vi "报表查询.vi"(11 "ConnectString":string="\"Provider=Microsoft.Jet.OLEDB.4.0;Data Source=C:\\\\Users\\\\Public\\\\Documents\\\\National \n\nInstruments\\\\TestStand 2017 (32-bit)\\\\Components\\\\Models\\\\TestStand Results.mdb;Persist Security Info=False\"") -> ()   [LabVIEW 2018, in "TestStand Simple UI.lvlib"]
uses:
  TestExec.llb/TestStand Simple UI.lvlib
  <vilib>/addons/database/Connection.llb/Conn ObjectReference.ctl
  <vilib>/addons/database/Connection.llb/DB Tools Open Connec (String).vi
  <vilib>/addons/database/Connection.llb/Conn Execute.vi
  <vilib>/addons/database/Recordset.llb/Rec Fetch Recordset Data (R).vi
  <vilib>/addons/database/Recordset.llb/Rec Destroy - Connection.vi
  <vilib>/Utility/file.llb/Write Delimited Spreadsheet (string).vi
  <vilib>/addons/database/_DB Variant To Data/Database Variant To Data.xnode
  <vilib>/addons/database/NI_Database_API.lvlib
panel:
  out "connection reference":T1
  out "error out":errorcluster
  in  "预览":bool
  in  "保存按钮":bool
  in  "搜索按钮":bool
  in  "二维码":string
  out "SN":string
  out "Row":i32
  in  "筛选结果":i32(listbox)
  in  "步骤结果":i32(listbox)
  in  "关键步骤":i32(listbox)
  out "data 2":string[][](array[string])
  out "tables":string[](array[string])
  in  "预览数据":i32(listbox)
  out "data 6":string[][](array[string])
  out "data 5":string[][](array[string])
  out "data 4":string[][](array[string])
  out "data 3":string[][](array[string])
  in  "测试报表":i32(listbox)
  out "data":string[][](array[string])
  in  "树形":string(tree)
  # "测试报表查询"
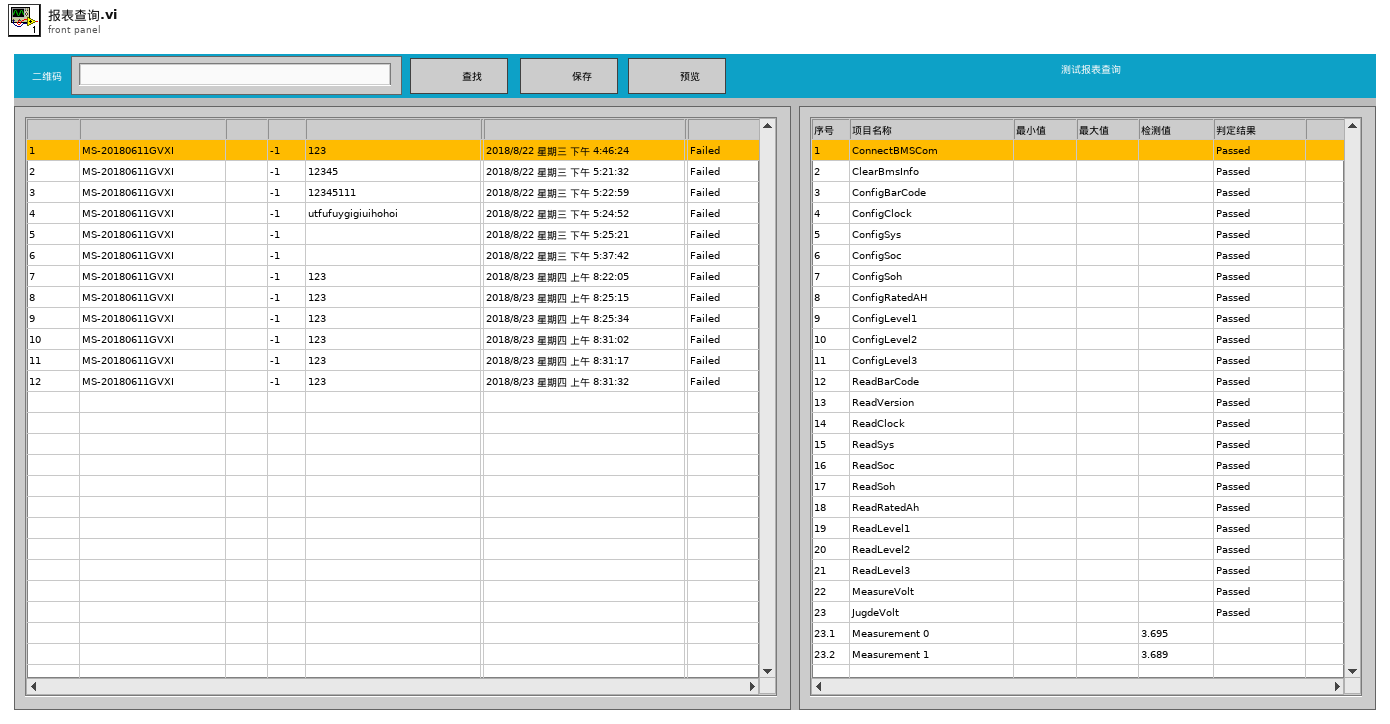
[diagram p1: front panel]
types:
  T1 = typedef "NI_Database_API.lvlib/Conn ObjectReference.ctl" = refnum<k1>
  T2 = typedef "LVPoint32TypeDef.ctl" = cluster{"Horizontal":i32, "Vertical":i32}
  T3 = typedef "LVRowAndColumnTypeDef.ctl" = cluster{"Row":i32, "Column":i32}
  T4 = typedef "NI_Database_API.lvlib/Rec ObjectReference.ctl" = refnum<k1>
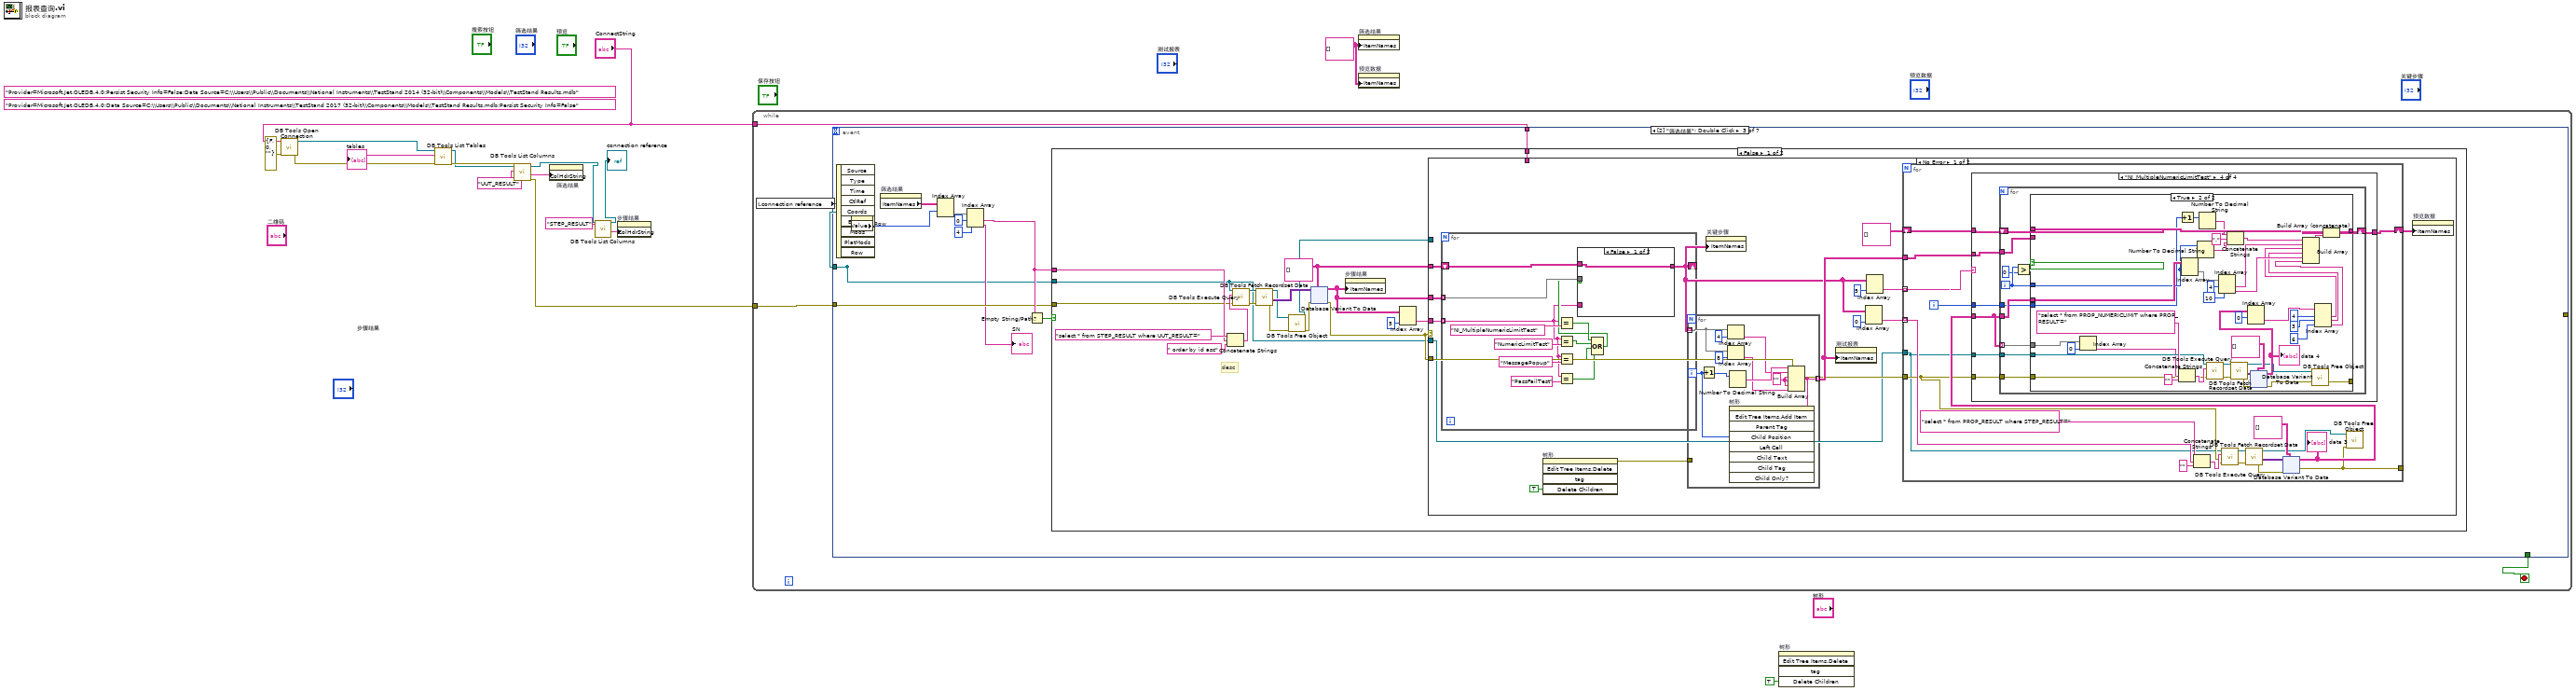
[diagram p0: block diagram]
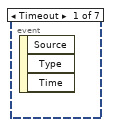
[diagram p2: hidden frame]
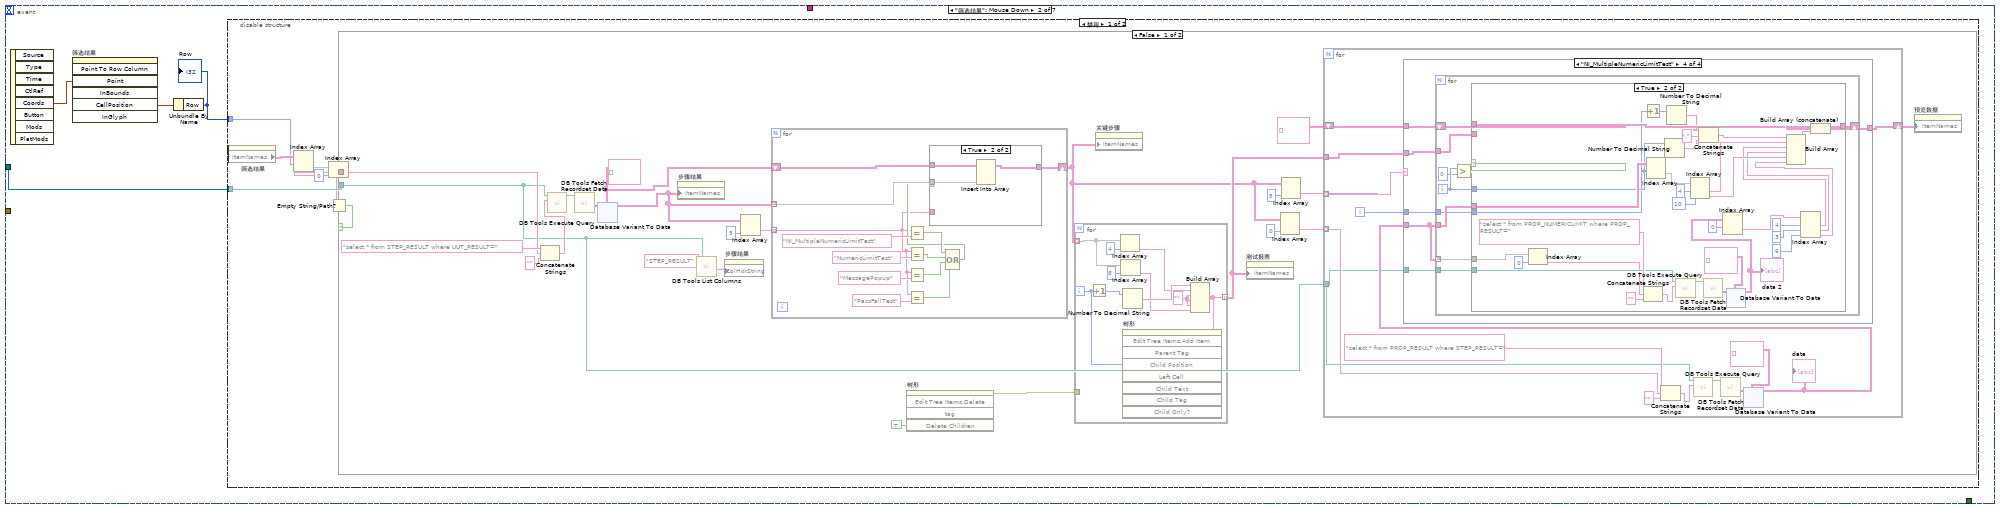
[diagram p3: hidden frame]
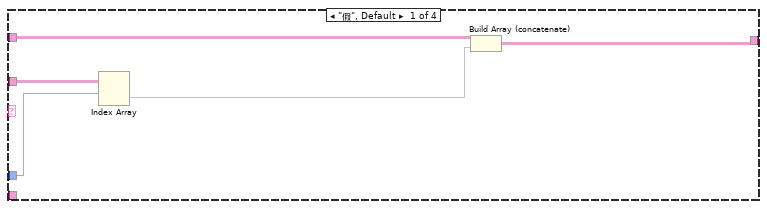
[diagram p4: hidden frame]
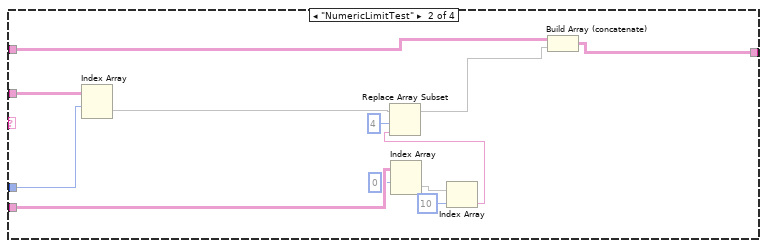
[diagram p5: hidden frame]
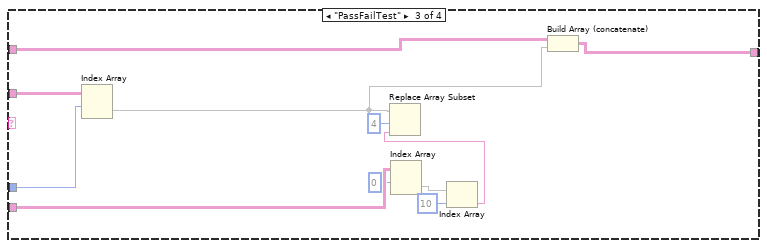
[diagram p6: hidden frame]
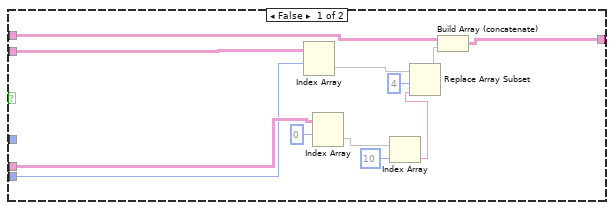
[diagram p7: hidden frame]
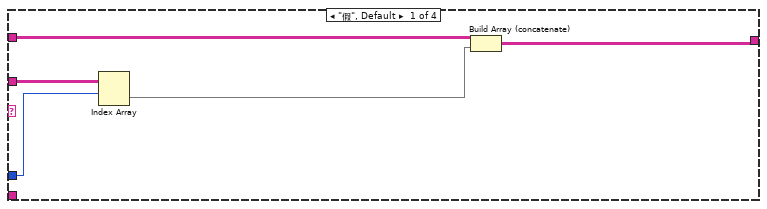
[diagram p11: hidden frame]
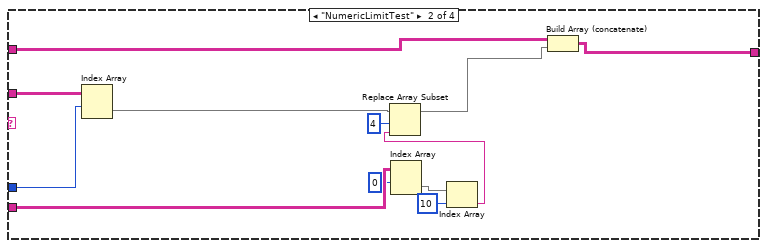
[diagram p12: hidden frame]
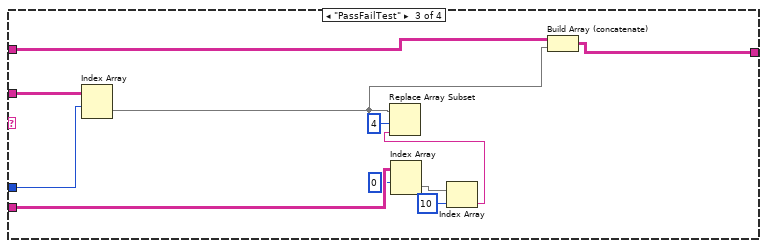
[diagram p13: hidden frame]
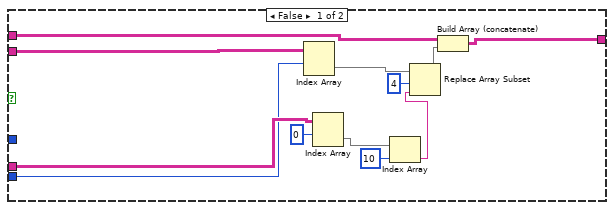
[diagram p14: hidden frame]
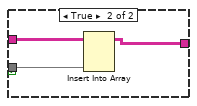
[diagram p15: hidden frame]
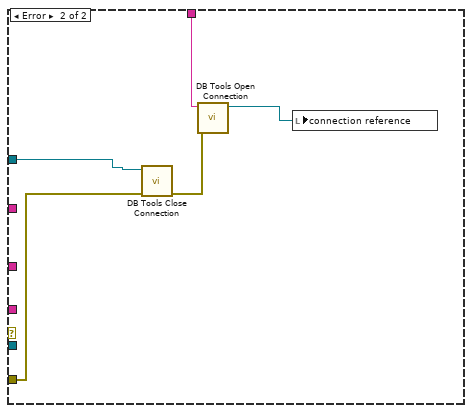
[diagram p16: hidden frame]
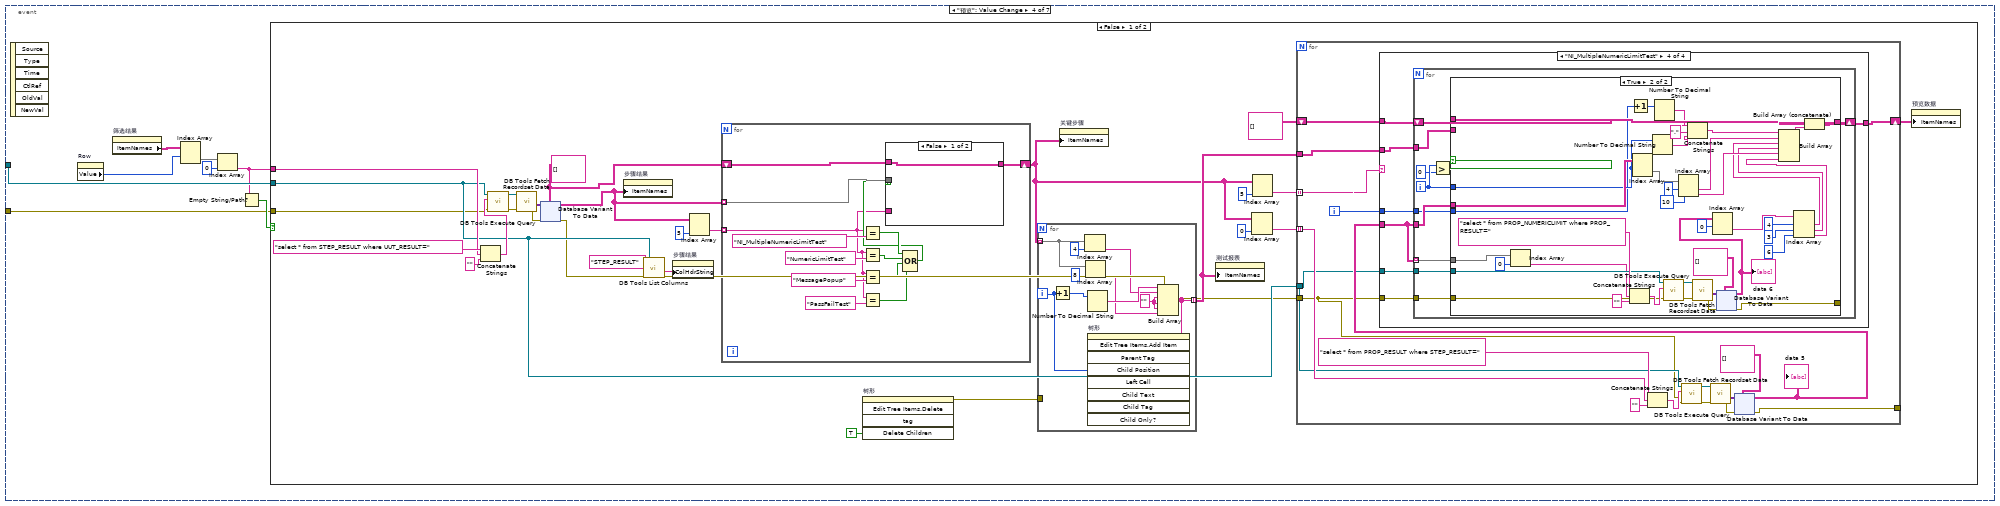
[diagram p18: hidden frame]
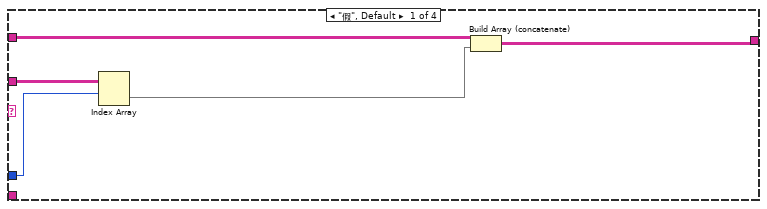
[diagram p19: hidden frame]
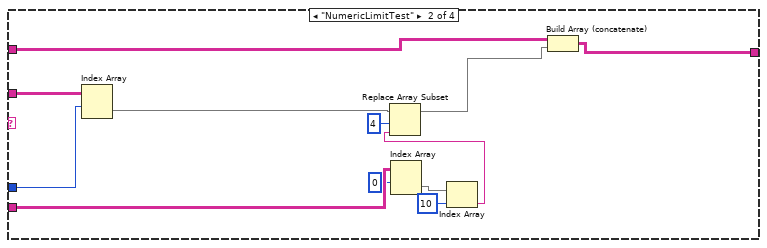
[diagram p20: hidden frame]
diagram:
  w1 = string[][] [] ("Item Names")
  (unwired) "Provider=Microsoft.Jet.OLEDB.4.0;Persist Security Info=False;Data Source=C:\\Users\\Public\\Documents\\National Instruments\\TestStand 2014 (32-bit)\\Components\\Models\\TestStand Results.mdb"
  (unwired) "Provider=Microsoft.Jet.OLEDB.4.0;Data Source=C:\\Users\\Public\\Documents\\National Instruments\\TestStand 2017 (32-bit)\\Components\\Models\\TestStand Results.mdb;Persist Security Info=False"
  n1 = call-poly <vilib>:"DB Tools Open Connection.vi"("error in (no error)"=errorcluster {"status"=FALSE, "code"=0, "source"=""}, "connection information"="ConnectString") -> ("error out"=w10:errorcluster, "connection reference"=w13:T1)  [unwired: 6 in]
  n2 = call <vilib>:"DB Tools List Tables.vi"("error in (no error)"=w10, "connection reference"=w13) -> ("error out"=w9:errorcluster, "tables"=→"tables":string[], "connection reference out"=w7:T1)  [unwired: 3 in]
  n3 = call <vilib>:"DB Tools List Columns.vi"("error in (no error)"=w9, "table"="UUT_RESULT", "connection reference"=w7) -> ("error out"=w8:errorcluster, "columns"=w14:string[], "connection reference out"=w4:T1)  [unwired: 1 in, 1 out]
  n4 = property on="筛选结果" class="MCListbox (strict)"("ColHdrString"=w14) -> ()  [unwired: 2 in, 2 out]
  n5 = call <vilib>:"DB Tools List Columns.vi"("table"="STEP_RESULT", "connection reference"=w4) -> ("columns"=w6:string[], "connection reference out"=→"connection reference":T1)  [unwired: 2 in, 2 out]
  n6 = property on="步骤结果" class="MCListbox (strict)"("ColHdrString"=w6) -> ()  [unwired: 2 in, 2 out]
  n7 = while {
    tunnel: w8 -> [w20]
    tunnel: "ConnectString" -> [w18]
    stop <- w19 stop-if-true
    n8 = local read "connection reference"() -> (w17:T1)
    n9 = event shown="[2] \"筛选结果\": Double Click" {
      selector: _ -> [_ _ _ _ _ _ _]
      dyn-events: _ -> [_ _ _ _ _ _ _]
      timeout: _ -> [_ _ _ _ _ _ _]
      tunnel: w17 -> [_ w22 w319 w649 _ w968 w973]
      tunnel: w20 -> [_ _ w323 w645 _ w967 w971]
      tunnel: [_ _ _ _ _ w969 _] -> w19
      tunnel: [_ _ _ _ _ _ w970] -> _
      tunnel: w18 -> [_ _ w320 _ _ _ _]
      tunnel: [_ _ w319 _ _ _ _] -> _
      event Timeout {
        n10 = event-data() -> ()  [unwired: 1 in, 3 out]
      }
      event "筛选结果": Mouse Down {
        n11 = event-data() -> ("Coords"=w24:T2)  [unwired: 1 in, 7 out]
        n12 = invoke on="筛选结果" class="MCListbox (严格)" method="Point To Row Column"("Point"=w24) -> ("CellPosition"=w23:T3)  [unwired: 6 in, 6 out]
        n13 = Unbundle By Name(w23) -> ("Row"=w21:i32)
        "Row" <- w21
        n14 = disable-structure shown="禁用" {
          disable-tunnel: w22 -> [w28 _]
          disable-tunnel: w21 -> [w27 _]
          frame Disabled {
            n15 = property on="筛选结果" class="MCListbox (strict)"() -> ("ItemNames"=w31:string[][])  [unwired: 2 in, 2 out]
            n16 = Index Array(array=w31, index (row)=w27) -> (element=w30:string[])  [unwired: 1 in]
            n17 = Index Array(array=w30, index=0 ("索引")) -> (element=w26:string)
            n18 = Empty String/Path?(string/path=w26) -> (empty?=w25:bool)
            n19 = case shown="False" w25 {
              tunnel: w28 -> [w36 _]
              tunnel: w26 -> [w48 _]
              frame False {
                w43 = string[][] []
                n20 = Concatenate Strings("select * from STEP_RESULT where UUT_RESULT=" ("condition"), w48, "" ("字符串")) -> (w50:string)
                n21 = call-poly <vilib>:"DB Tools Execute Query.vi"("SQL query"=w50, "connection reference"=w36) -> ("recordset reference"=w54:T4)  [unwired: 6 in, 1 out]
                n22 = call-poly <vilib>:"DB Tools Fetch Recordset Data.vi"("recordset reference"=w54) -> ("recordset data"=w53:variant[][])  [unwired: 4 in, 2 out]
                n23 = xnode "Database Variant To Data"("database variant"=w53, "type"=w43) -> ("data"=w44:string[][])  [unwired: 1 in, 1 out]
                n24 = property on="步骤结果" class="MCListbox (strict)"("ItemNames"=w44) -> ()  [unwired: 2 in, 2 out]
                n25 = call <vilib>:"DB Tools List Columns.vi"("table"="STEP_RESULT", "connection reference"=w36) -> ("columns"=w47:string[])  [unwired: 2 in, 3 out]
                n26 = property on="步骤结果" class="MCListbox (strict)"("ColHdrString"=w47) -> ()  [unwired: 2 in, 2 out]
                n27 = Index Array(array=w44, index (col)=5 ("禁用的索引 (列)")) -> (element=w45:string[])  [unwired: 1 in]
                n28 = for {
                  tunnel: w45 -> [w259] mode=indexing
                  tunnel: w44 -> [w263] mode=indexing
                  shift-right: [w261] -> w38
                  shift-left: w43 -> [w264]
                  n29 = Equal?(x=w259, y="NI_MultipleNumericLimitTest") -> (x = y?=w267:bool)
                  n30 = Equal?(x=w259, y="NumericLimitTest") -> (x = y?=w266:bool)
                  n31 = Equal?(x=w259, y="MessagePopup") -> (x = y?=w265:bool)
                  n32 = Equal?(x=w259, y="PassFailTest") -> (x = y?=w258:bool)
                  n33 = Compound Arithmetic op=OR(w267, w266, w265, w258) -> (w262:bool)
                  n34 = case shown="True" w262 {
                    tunnel: w264 -> [w271 w274]
                    tunnel: w263 -> [_ w273]
                    tunnel: [w271 w272] -> w261
                    tunnel: w259 -> [_ _]
                    frame False {
                    }
                    frame True {
                      n35 = Insert Into Array(array=w274, new element=w273) -> (w272:string[][])  [unwired: 2 in]
                    }
                  }
                }
                n36 = invoke on="树形" class="Tree (严格)" method="Edit Tree Items.Delete"("Delete Children"=TRUE ("删除子项？")) -> (error out=w34:errorcluster)  [unwired: 4 in, 4 out]
                n37 = for {
                  tunnel: w38 -> [w253] mode=indexing
                  tunnel: [w249] -> w42 mode=indexing
                  tunnel: w34 -> [_]
                  i -> [w248]
                  w251 = ""
                  n38 = Increment(x=w248) -> (x+1=w257:i32)
                  n39 = Index Array(array=w253, index=4 ("索引")) -> (element=w254:string)
                  n40 = Index Array(array=w253, index=8 ("索引")) -> (element=w250:string)
                  n41 = Number To Decimal String(number=w257) -> (decimal integer string=w256:string)  [unwired: 1 in]
                  n42 = Build Array(w256, w254, w251, w251, w251, w250) -> (w249:string[])
                  n43 = invoke on="树形" class="Tree (严格)" method="Edit Tree Items.Add Item"("Child Position"=w248, "Child Text"=w249) -> ()  [unwired: 7 in, 9 out]
                }
                n44 = property on="关键步骤" class="MCListbox (strict)"("ItemNames"=w38) -> ()  [unwired: 2 in, 2 out]
                n45 = property on="测试报表" class="MCListbox (strict)"("ItemNames"=w42) -> ()  [unwired: 2 in, 2 out]
                n46 = Index Array(array=w38, index (col)=0 ("禁用的索引 (列)")) -> (element=w37:string[])  [unwired: 1 in]
                n47 = Index Array(array=w38, index (col)=5 ("禁用的索引 (列)")) -> (element=w40:string[])  [unwired: 1 in]
                n48 = for {
                  tunnel: w40 -> [w68] mode=indexing
                  tunnel: w37 -> [w61] mode=indexing
                  tunnel: w36 -> [w55]
                  shift-right: [w57] -> w32
                  shift-left: string[][] [] -> [w58]
                  tunnel: w42 -> [w60]
                  i -> [w59]
                  n49 = Concatenate Strings("select * from PROP_RESULT where STEP_RESULT=" ("condition"), w61, "" ("字符串")) -> (w64:string)
                  n50 = call-poly <vilib>:"DB Tools Execute Query.vi"("SQL query"=w64, "connection reference"=w55) -> ("recordset reference"=w67:T4)  [unwired: 6 in, 1 out]
                  n51 = call-poly <vilib>:"DB Tools Fetch Recordset Data.vi"("recordset reference"=w67) -> ("recordset data"=w66:variant[][])  [unwired: 4 in, 2 out]
                  n52 = xnode "Database Variant To Data"("database variant"=w66, "type"=string[][] []) -> ("data"=w56:string[][])  [unwired: 1 in, 1 out]
                  "data" <- w56
                  n53 = case shown="\"NI_MultipleNumericLimitTest\"" w68 {
                    tunnel: w60 -> [w116 w122 w134 w142]
                    tunnel: w59 -> [w113 w121 w133 w146]
                    tunnel: w56 -> [_ w127 w139 w144]
                    tunnel: w58 -> [w117 w120 w132 w143]
                    tunnel: [w114 w118 w131 w145] -> w57
                    tunnel: w55 -> [_ _ _ w141]
                    frame "假", Default {
                      n54 = Index Array(array=w116, index (row)=w113) -> (element=w115:string[])  [unwired: 1 in]
                      n55 = Build Array (concatenate)(w117, w115) -> (w114:string[][])
                    }
                    frame "NumericLimitTest" {
                      n56 = Index Array(array=w122, index (row)=w121) -> (element=w129:string[])  [unwired: 1 in]
                      n57 = Index Array(array=w127, index (row)=0 ("索引 (行)")) -> (element=w125:string[])  [unwired: 1 in]
                      n58 = Index Array(array=w125, index=10 ("索引")) -> (element=w123:string)
                      n59 = Replace Array Subset(array=w129, new element=w123, index=4 ("索引")) -> (w119:string[])
                      n60 = Build Array (concatenate)(w120, w119) -> (w118:string[][])
                    }
                    frame "PassFailTest" {
                      n61 = Index Array(array=w134, index (row)=w133) -> (element=w130:string[])  [unwired: 1 in]
                      n62 = Index Array(array=w139, index (row)=0 ("索引 (行)")) -> (element=w137:string[])  [unwired: 1 in]
                      n63 = Index Array(array=w137, index=10 ("索引")) -> (element=w135:string)
                      n64 = Replace Array Subset(array=w130, new element=w135, index=4 ("索引")) -> ()  [unwired: 1 out]
                      n65 = Build Array (concatenate)(w132, w130) -> (w131:string[][])
                    }
                    frame "NI_MultipleNumericLimitTest" {
                      n66 = for {
                        tunnel: w144 -> [w156]
                        tunnel: w142 -> [w155]
                        tunnel: w146 -> [w154]
                        shift-right: [w152] -> w145
                        shift-left: w143 -> [w153]
                        tunnel: w144 -> [w147] mode=indexing
                        tunnel: w141 -> [w148]
                        i -> [w151]
                        n67 = Greater?(x=w151, y=0) -> (0:w150:bool)
                        n68 = case shown="True" w150 {
                          tunnel: w156 -> [w166 w200]
                          tunnel: w155 -> [w168 _]
                          tunnel: w154 -> [w165 w188]
                          tunnel: w153 -> [w159 w202]
                          tunnel: [w157 w201] -> w152
                          tunnel: w151 -> [_ w198]
                          tunnel: w148 -> [_ w181]
                          tunnel: w147 -> [_ w180]
                          frame False {
                            n69 = Index Array(array=w168, index (row)=w165) -> (element=w167:string[])  [unwired: 1 in]
                            n70 = Index Array(array=w166, index (row)=0 ("索引 (行)")) -> (element=w163:string[])  [unwired: 1 in]
                            n71 = Index Array(array=w163, index=10 ("索引")) -> (element=w160:string)
                            n72 = Replace Array Subset(array=w167, new element=w160, index=4 ("索引")) -> (w158:string[])
                            n73 = Build Array (concatenate)(w159, w158) -> (w157:string[][])
                          }
                          frame True {
                            n74 = Index Array(array=w180, index=0 ("索引")) -> (element=w178:string)
                            n75 = Concatenate Strings("select * from PROP_NUMERICLIMIT where PROP_RESULT=" ("condition"), w178, "" ("字符串")) -> (w185:string)
                            n76 = Increment(x=w188) -> (x+1=w189:i32)
                            n77 = Index Array(array=w200, index (row)=w198) -> (element=w199:string[])  [unwired: 1 in]
                            n78 = Number To Decimal String(number=w198) -> (decimal integer string=w191:string)  [unwired: 1 in]
                            n79 = Number To Decimal String(number=w189) -> (decimal integer string=w193:string)  [unwired: 1 in]
                            n80 = call-poly <vilib>:"DB Tools Execute Query.vi"("SQL query"=w185, "connection reference"=w181) -> ("recordset reference"=w182:T4)  [unwired: 6 in, 1 out]
                            n81 = Index Array(array=w199, index #1=4 ("索引"), index #2=10 ("索引")) -> (element #1=w196:string, element #2=w195:string)
                            n82 = Concatenate Strings(w193, "." ("字符串"), w191) -> (w190:string)
                            n83 = call-poly <vilib>:"DB Tools Fetch Recordset Data.vi"("recordset reference"=w182) -> ("recordset data"=w183:variant[][])  [unwired: 4 in, 2 out]
                            n84 = xnode "Database Variant To Data"("database variant"=w183, "type"=string[][] []) -> ("data"=w176:string[][])  [unwired: 1 in, 1 out]
                            "data 2" <- w176
                            n85 = Index Array(array=w176, index (row)=0 ("索引")) -> (element=w175:string[])  [unwired: 1 in]
                            n86 = Index Array(array=w175, index #1=4 ("索引"), index #2=3 ("索引"), index #3=6 ("索引")) -> (element #1=w171:string, element #2=w170:string, element #3=w169:string)
                            n87 = Build Array(w190, w196, w171, w170, w195, w169) -> (w194:string[])
                            n88 = Build Array (concatenate)(w202, w194) -> (w201:string[][])
                          }
                        }
                      }
                    }
                  }
                }
                n89 = property on="预览数据" class="MCListbox (strict)"("ItemNames"=w32) -> ()  [unwired: 2 in, 2 out]
              }
              frame True {
              }
            }
          }
          frame Enabled {
          }
        }
      }
      event "筛选结果": Double Click {
        n90 = event-data() -> ()  [unwired: 1 in, 9 out]
        n91 = property on="Row" class="DigNum (strict)"() -> ("Value"=w324:i32)  [unwired: 2 in, 2 out]
        n92 = property on="筛选结果" class="MCListbox (strict)"() -> ("ItemNames"=w329:string[][])  [unwired: 2 in, 2 out]
        n93 = Index Array(array=w329, index (row)=w324) -> (element=w328:string[])  [unwired: 1 in]
        n94 = Index Array(array=w328, index #1=0 ("索引"), index #2=4 ("索引")) -> (element #1=w326:string, element #2=→"SN":string)
        n95 = Empty String/Path?(string/path=w326) -> (empty?=w325:bool)
        n96 = case shown="False" w325 {
          tunnel: w319 -> [w334 _]
          tunnel: w326 -> [w343 _]
          tunnel: w323 -> [w335 _]
          tunnel: w320 -> [w337 _]
          frame False {
            w339 = string[][] []
            # "desc"
            n97 = Concatenate Strings("select * from STEP_RESULT where UUT_RESULT=" ("condition"), w343, " order by id asc" ("字符串")) -> (w344:string)
            n98 = call-poly <vilib>:"DB Tools Execute Query.vi"("error in (no error)"=w335, "SQL query"=w344, "connection reference"=w334) -> ("error out"=w338:errorcluster, "recordset reference"=w348:T4)  [unwired: 5 in]
            n99 = call-poly <vilib>:"DB Tools Fetch Recordset Data.vi"("error in (no error)"=w338, "recordset reference"=w348) -> ("error out"=w332:errorcluster, "recordset data"=w347:variant[][], "recordset reference out"=w333:T4)  [unwired: 3 in]
            n100 = call-poly <vilib>:"DB Tools Free Object.vi"("error in (no error)"=w332, "recordset reference"=w333) -> ("error out"=w331:errorcluster, "connection reference"=w330:T1)  [unwired: 8 in]
            n101 = xnode "Database Variant To Data"("database variant"=w347, "error in (no error)"=w331, "type"=w339) -> ("data"=w340:string[][], "error out"=w336:errorcluster)
            n102 = property on="步骤结果" class="MCListbox (strict)"("ItemNames"=w340) -> ()  [unwired: 2 in, 2 out]
            n103 = Index Array(array=w340, index (col)=5 ("禁用的索引 (列)")) -> (element=w341:string[])  [unwired: 1 in]
            n104 = case shown="No Error" w336 {
              tunnel: w341 -> [w363 _]
              tunnel: w340 -> [w362 _]
              tunnel: w339 -> [w361 _]
              tunnel: w336 -> [w350 w596]
              tunnel: w337 -> [_ w600]
              tunnel: w334 -> [w349 _]
              tunnel: w330 -> [_ w597]
              frame No Error {
                n105 = for {
                  tunnel: w363 -> [w580] mode=indexing
                  tunnel: w362 -> [w584] mode=indexing
                  shift-right: [w582] -> w356
                  shift-left: w361 -> [w585]
                  n106 = Equal?(x=w580, y="NI_MultipleNumericLimitTest") -> (x = y?=w588:bool)
                  n107 = Equal?(x=w580, y="NumericLimitTest") -> (x = y?=w587:bool)
                  n108 = Equal?(x=w580, y="MessagePopup") -> (x = y?=w586:bool)
                  n109 = Equal?(x=w580, y="PassFailTest") -> (x = y?=w579:bool)
                  n110 = Compound Arithmetic op=OR(w588, w587, w586, w579) -> (w583:bool)
                  n111 = case shown="False" w583 {
                    tunnel: w585 -> [w592 w595]
                    tunnel: w584 -> [_ w594]
                    tunnel: [w592 w593] -> w582
                    tunnel: w580 -> [_ _]
                    frame False {
                    }
                    frame True {
                      n112 = Insert Into Array(array=w595, new element=w594) -> (w593:string[][])  [unwired: 2 in]
                    }
                  }
                }
                n113 = invoke on="树形" class="Tree (严格)" method="Edit Tree Items.Delete"("Delete Children"=TRUE ("删除子项？")) -> (error out=w353:errorcluster)  [unwired: 4 in, 4 out]
                n114 = for {
                  tunnel: w356 -> [w574] mode=indexing
                  tunnel: [w570] -> w360 mode=indexing
                  tunnel: w353 -> [_]
                  i -> [w569]
                  w572 = ""
                  n115 = Increment(x=w569) -> (x+1=w578:i32)
                  n116 = Index Array(array=w574, index=4 ("索引")) -> (element=w575:string)
                  n117 = Index Array(array=w574, index=8 ("索引")) -> (element=w571:string)
                  n118 = Number To Decimal String(number=w578) -> (decimal integer string=w577:string)  [unwired: 1 in]
                  n119 = Build Array(w577, w575, w572, w572, w572, w571) -> (w570:string[])
                  n120 = invoke on="树形" class="Tree (严格)" method="Edit Tree Items.Add Item"("Child Position"=w569, "Child Text"=w570) -> ()  [unwired: 7 in, 9 out]
                }
                n121 = property on="关键步骤" class="MCListbox (strict)"("ItemNames"=w356) -> ()  [unwired: 2 in, 2 out]
                n122 = property on="测试报表" class="MCListbox (strict)"("ItemNames"=w360) -> ()  [unwired: 2 in, 2 out]
                n123 = Index Array(array=w356, index (col)=0 ("禁用的索引 (列)")) -> (element=w355:string[])  [unwired: 1 in]
                n124 = Index Array(array=w356, index (col)=5 ("禁用的索引 (列)")) -> (element=w358:string[])  [unwired: 1 in]
                n125 = for {
                  tunnel: w358 -> [w382] mode=indexing
                  tunnel: w355 -> [w375] mode=indexing
                  tunnel: w349 -> [w364]
                  shift-right: [w371] -> w351
                  shift-left: string[][] [] -> [w372]
                  tunnel: w360 -> [w374]
                  tunnel: w350 -> [w369]
                  tunnel: [w365] -> _
                  i -> [w373]
                  n126 = Concatenate Strings("select * from PROP_RESULT where STEP_RESULT=" ("condition"), w375, "" ("字符串")) -> (w378:string)
                  n127 = call-poly <vilib>:"DB Tools Execute Query.vi"("error in (no error)"=w369, "SQL query"=w378, "connection reference"=w364) -> ("error out"=w368:errorcluster, "recordset reference"=w381:T4)  [unwired: 5 in]
                  n128 = call-poly <vilib>:"DB Tools Fetch Recordset Data.vi"("error in (no error)"=w368, "recordset reference"=w381) -> ("error out"=w367:errorcluster, "recordset data"=w380:variant[][], "recordset reference out"=w366:T4)  [unwired: 3 in]
                  n129 = xnode "Database Variant To Data"("database variant"=w380, "error in (no error)"=w367, "type"=string[][] []) -> ("data"=w370:string[][], "error out"=w365:errorcluster)
                  "data 3" <- w370
                  n130 = case shown="\"NI_MultipleNumericLimitTest\"" w382 {
                    tunnel: w374 -> [w430 w436 w448 w457]
                    tunnel: w373 -> [w427 w435 w447 w461]
                    tunnel: w370 -> [_ w441 w453 w459]
                    tunnel: w372 -> [w431 w434 w446 w458]
                    tunnel: [w428 w432 w445 w460] -> w371
                    tunnel: w364 -> [_ _ _ w456]
                    tunnel: w369 -> [_ _ _ w455]
                    frame "假", Default {
                      n131 = Index Array(array=w430, index (row)=w427) -> (element=w429:string[])  [unwired: 1 in]
                      n132 = Build Array (concatenate)(w431, w429) -> (w428:string[][])
                    }
                    frame "NumericLimitTest" {
                      n133 = Index Array(array=w436, index (row)=w435) -> (element=w443:string[])  [unwired: 1 in]
                      n134 = Index Array(array=w441, index (row)=0 ("索引 (行)")) -> (element=w439:string[])  [unwired: 1 in]
                      n135 = Index Array(array=w439, index=10 ("索引")) -> (element=w437:string)
                      n136 = Replace Array Subset(array=w443, new element=w437, index=4 ("索引")) -> (w433:string[])
                      n137 = Build Array (concatenate)(w434, w433) -> (w432:string[][])
                    }
                    frame "PassFailTest" {
                      n138 = Index Array(array=w448, index (row)=w447) -> (element=w444:string[])  [unwired: 1 in]
                      n139 = Index Array(array=w453, index (row)=0 ("索引 (行)")) -> (element=w451:string[])  [unwired: 1 in]
                      n140 = Index Array(array=w451, index=10 ("索引")) -> (element=w449:string)
                      n141 = Replace Array Subset(array=w444, new element=w449, index=4 ("索引")) -> ()  [unwired: 1 out]
                      n142 = Build Array (concatenate)(w446, w444) -> (w445:string[][])
                    }
                    frame "NI_MultipleNumericLimitTest" {
                      n143 = for {
                        tunnel: w459 -> [w472]
                        tunnel: w457 -> [w471]
                        tunnel: w461 -> [w470]
                        shift-right: [w468] -> w460
                        shift-left: w458 -> [w469]
                        tunnel: w459 -> [w463] mode=indexing
                        tunnel: w456 -> [w464]
                        tunnel: w455 -> [w462]
                        i -> [w467]
                        n144 = Greater?(x=w467, y=0) -> (0:w466:bool)
                        n145 = case shown="True" w466 {
                          tunnel: w472 -> [w482 w521]
                          tunnel: w471 -> [w484 _]
                          tunnel: w470 -> [w481 w509]
                          tunnel: w469 -> [w475 w523]
                          tunnel: [w473 w522] -> w468
                          tunnel: w467 -> [_ w519]
                          tunnel: w464 -> [_ w502]
                          tunnel: w463 -> [_ w501]
                          tunnel: w462 -> [_ w489]
                          tunnel: [_ w486] -> _
                          frame False {
                            n146 = Index Array(array=w484, index (row)=w481) -> (element=w483:string[])  [unwired: 1 in]
                            n147 = Index Array(array=w482, index (row)=0 ("索引 (行)")) -> (element=w479:string[])  [unwired: 1 in]
                            n148 = Index Array(array=w479, index=10 ("索引")) -> (element=w476:string)
                            n149 = Replace Array Subset(array=w483, new element=w476, index=4 ("索引")) -> (w474:string[])
                            n150 = Build Array (concatenate)(w475, w474) -> (w473:string[][])
                          }
                          frame True {
                            n151 = Index Array(array=w501, index=0 ("索引")) -> (element=w499:string)
                            n152 = Concatenate Strings("select * from PROP_NUMERICLIMIT where PROP_RESULT=" ("condition"), w499, "" ("字符串")) -> (w506:string)
                            n153 = Increment(x=w509) -> (x+1=w510:i32)
                            n154 = Index Array(array=w521, index (row)=w519) -> (element=w520:string[])  [unwired: 1 in]
                            n155 = Number To Decimal String(number=w519) -> (decimal integer string=w512:string)  [unwired: 1 in]
                            n156 = Number To Decimal String(number=w510) -> (decimal integer string=w514:string)  [unwired: 1 in]
                            n157 = call-poly <vilib>:"DB Tools Execute Query.vi"("error in (no error)"=w489, "SQL query"=w506, "connection reference"=w502) -> ("error out"=w488:errorcluster, "recordset reference"=w503:T4)  [unwired: 5 in]
                            n158 = Index Array(array=w520, index #1=4 ("索引"), index #2=10 ("索引")) -> (element #1=w517:string, element #2=w516:string)
                            n159 = Concatenate Strings(w514, "." ("字符串"), w512) -> (w511:string)
                            n160 = call-poly <vilib>:"DB Tools Fetch Recordset Data.vi"("error in (no error)"=w488, "recordset reference"=w503) -> ("error out"=w487:errorcluster, "recordset data"=w504:variant[][], "recordset reference out"=w485:T4)  [unwired: 3 in]
                            n161 = xnode "Database Variant To Data"("database variant"=w504, "error in (no error)"=w487, "type"=string[][] []) -> ("data"=w497:string[][], "error out"=w486:errorcluster)
                            "data 4" <- w497
                            n162 = Index Array(array=w497, index (row)=0 ("索引")) -> (element=w496:string[])  [unwired: 1 in]
                            n163 = call-poly <vilib>:"DB Tools Free Object.vi"("recordset reference"=w485) -> ()  [unwired: 9 in, 2 out]
                            n164 = Index Array(array=w496, index #1=4 ("索引"), index #2=3 ("索引"), index #3=6 ("索引")) -> (element #1=w492:string, element #2=w491:string, element #3=w490:string)
                            n165 = Build Array(w511, w517, w492, w491, w516, w490) -> (w515:string[])
                            n166 = Build Array (concatenate)(w523, w515) -> (w522:string[][])
                          }
                        }
                      }
                    }
                  }
                  n167 = call-poly <vilib>:"DB Tools Free Object.vi"("error in (no error)"=w365, "recordset reference"=w366) -> ()  [unwired: 8 in, 2 out]
                }
                n168 = property on="预览数据" class="MCListbox (strict)"("ItemNames"=w351) -> ()  [unwired: 2 in, 2 out]
              }
              frame Error {
                n169 = call <vilib>:"DB Tools Close Connection.vi"("error in (no error)"=w596, "connection reference"=w597) -> ("error out"=w598:errorcluster)  [unwired: 5 in]
                n170 = call-poly <vilib>:"DB Tools Open Connection.vi"("error in (no error)"=w598, "connection information"=w600) -> ("connection reference"=w599:T1)  [unwired: 6 in, 1 out]
                n171 = local write "connection reference"(w599) -> ()
              }
            }
          }
          frame True {
          }
        }
      }
      event "预览": Value Change {
        n172 = event-data() -> ()  [unwired: 1 in, 6 out]
        n173 = property on="Row" class="DigNum (strict)"() -> ("Value"=w646:i32)  [unwired: 2 in, 2 out]
        n174 = property on="筛选结果" class="MCListbox (strict)"() -> ("ItemNames"=w652:string[][])  [unwired: 2 in, 2 out]
        n175 = Index Array(array=w652, index (row)=w646) -> (element=w651:string[])  [unwired: 1 in]
        n176 = Index Array(array=w651, index=0 ("索引")) -> (element=w648:string)
        n177 = Empty String/Path?(string/path=w648) -> (empty?=w647:bool)
        n178 = case shown="False" w647 {
          tunnel: w649 -> [w662 _]
          tunnel: w648 -> [w674 _]
          tunnel: w645 -> [w657 _]
          frame False {
            w669 = string[][] []
            n179 = Concatenate Strings("select * from STEP_RESULT where UUT_RESULT=" ("condition"), w674, "" ("字符串")) -> (w676:string)
            n180 = call-poly <vilib>:"DB Tools Execute Query.vi"("error in (no error)"=w657, "SQL query"=w676, "connection reference"=w662) -> ("error out"=w656:errorcluster, "recordset reference"=w680:T4)  [unwired: 5 in]
            n181 = call-poly <vilib>:"DB Tools Fetch Recordset Data.vi"("error in (no error)"=w656, "recordset reference"=w680) -> ("error out"=w655:errorcluster, "recordset data"=w679:variant[][])  [unwired: 3 in, 1 out]
            n182 = xnode "Database Variant To Data"("database variant"=w679, "error in (no error)"=w655, "type"=w669) -> ("data"=w670:string[][], "error out"=w654:errorcluster)
            n183 = property on="步骤结果" class="MCListbox (strict)"("ItemNames"=w670) -> ()  [unwired: 2 in, 2 out]
            n184 = call <vilib>:"DB Tools List Columns.vi"("error in (no error)"=w654, "table"="STEP_RESULT", "connection reference"=w662) -> ("error out"=w653:errorcluster, "columns"=w673:string[])  [unwired: 1 in, 2 out]
            n185 = property on="步骤结果" class="MCListbox (strict)"("ColHdrString"=w673) -> ()  [unwired: 2 in, 2 out]
            n186 = Index Array(array=w670, index (col)=5 ("禁用的索引 (列)")) -> (element=w671:string[])  [unwired: 1 in]
            n187 = for {
              tunnel: w671 -> [w895] mode=indexing
              tunnel: w670 -> [w899] mode=indexing
              shift-right: [w897] -> w664
              shift-left: w669 -> [w900]
              n188 = Equal?(x=w895, y="NI_MultipleNumericLimitTest") -> (x = y?=w903:bool)
              n189 = Equal?(x=w895, y="NumericLimitTest") -> (x = y?=w902:bool)
              n190 = Equal?(x=w895, y="MessagePopup") -> (x = y?=w901:bool)
              n191 = Equal?(x=w895, y="PassFailTest") -> (x = y?=w894:bool)
              n192 = Compound Arithmetic op=OR(w903, w902, w901, w894) -> (w898:bool)
              n193 = case shown="False" w898 {
                tunnel: w900 -> [w907 w910]
                tunnel: w899 -> [_ w909]
                tunnel: [w907 w908] -> w897
                tunnel: w895 -> [_ _]
                frame False {
                }
                frame True {
                  n194 = Insert Into Array(array=w910, new element=w909) -> (w908:string[][])  [unwired: 2 in]
                }
              }
            }
            n195 = invoke on="树形" class="Tree (严格)" method="Edit Tree Items.Delete"("Delete Children"=TRUE ("删除子项？")) -> (error out=w660:errorcluster)  [unwired: 4 in, 4 out]
            n196 = for {
              tunnel: w664 -> [w889] mode=indexing
              tunnel: [w885] -> w668 mode=indexing
              tunnel: w660 -> [_]
              i -> [w884]
              w887 = ""
              n197 = Increment(x=w884) -> (x+1=w893:i32)
              n198 = Index Array(array=w889, index=4 ("索引")) -> (element=w890:string)
              n199 = Index Array(array=w889, index=8 ("索引")) -> (element=w886:string)
              n200 = Number To Decimal String(number=w893) -> (decimal integer string=w892:string)  [unwired: 1 in]
              n201 = Build Array(w892, w890, w887, w887, w887, w886) -> (w885:string[])
              n202 = invoke on="树形" class="Tree (严格)" method="Edit Tree Items.Add Item"("Child Position"=w884, "Child Text"=w885) -> ()  [unwired: 7 in, 9 out]
            }
            n203 = property on="关键步骤" class="MCListbox (strict)"("ItemNames"=w664) -> ()  [unwired: 2 in, 2 out]
            n204 = property on="测试报表" class="MCListbox (strict)"("ItemNames"=w668) -> ()  [unwired: 2 in, 2 out]
            n205 = Index Array(array=w664, index (col)=0 ("禁用的索引 (列)")) -> (element=w663:string[])  [unwired: 1 in]
            n206 = Index Array(array=w664, index (col)=5 ("禁用的索引 (列)")) -> (element=w666:string[])  [unwired: 1 in]
            n207 = for {
              tunnel: w666 -> [w698] mode=indexing
              tunnel: w663 -> [w691] mode=indexing
              tunnel: w662 -> [w685]
              shift-right: [w687] -> w658
              shift-left: string[][] [] -> [w688]
              tunnel: w668 -> [w690]
              tunnel: w653 -> [w684]
              tunnel: [w681] -> _
              i -> [w689]
              n208 = Concatenate Strings("select * from PROP_RESULT where STEP_RESULT=" ("condition"), w691, "" ("字符串")) -> (w694:string)
              n209 = call-poly <vilib>:"DB Tools Execute Query.vi"("error in (no error)"=w684, "SQL query"=w694, "connection reference"=w685) -> ("error out"=w683:errorcluster, "recordset reference"=w697:T4)  [unwired: 5 in]
              n210 = call-poly <vilib>:"DB Tools Fetch Recordset Data.vi"("error in (no error)"=w683, "recordset reference"=w697) -> ("error out"=w682:errorcluster, "recordset data"=w696:variant[][])  [unwired: 3 in, 1 out]
              n211 = xnode "Database Variant To Data"("database variant"=w696, "error in (no error)"=w682, "type"=string[][] []) -> ("data"=w686:string[][], "error out"=w681:errorcluster)
              "data 5" <- w686
              n212 = case shown="\"NI_MultipleNumericLimitTest\"" w698 {
                tunnel: w690 -> [w746 w752 w764 w773]
                tunnel: w689 -> [w743 w751 w763 w777]
                tunnel: w686 -> [_ w757 w769 w775]
                tunnel: w688 -> [w747 w750 w762 w774]
                tunnel: [w744 w748 w761 w776] -> w687
                tunnel: w685 -> [_ _ _ w772]
                tunnel: w684 -> [_ _ _ w771]
                frame "假", Default {
                  n213 = Index Array(array=w746, index (row)=w743) -> (element=w745:string[])  [unwired: 1 in]
                  n214 = Build Array (concatenate)(w747, w745) -> (w744:string[][])
                }
                frame "NumericLimitTest" {
                  n215 = Index Array(array=w752, index (row)=w751) -> (element=w759:string[])  [unwired: 1 in]
                  n216 = Index Array(array=w757, index (row)=0 ("索引 (行)")) -> (element=w755:string[])  [unwired: 1 in]
                  n217 = Index Array(array=w755, index=10 ("索引")) -> (element=w753:string)
                  n218 = Replace Array Subset(array=w759, new element=w753, index=4 ("索引")) -> (w749:string[])
                  n219 = Build Array (concatenate)(w750, w749) -> (w748:string[][])
                }
                frame "PassFailTest" {
                  n220 = Index Array(array=w764, index (row)=w763) -> (element=w760:string[])  [unwired: 1 in]
                  n221 = Index Array(array=w769, index (row)=0 ("索引 (行)")) -> (element=w767:string[])  [unwired: 1 in]
                  n222 = Index Array(array=w767, index=10 ("索引")) -> (element=w765:string)
                  n223 = Replace Array Subset(array=w760, new element=w765, index=4 ("索引")) -> ()  [unwired: 1 out]
                  n224 = Build Array (concatenate)(w762, w760) -> (w761:string[][])
                }
                frame "NI_MultipleNumericLimitTest" {
                  n225 = for {
                    tunnel: w775 -> [w788]
                    tunnel: w773 -> [w787]
                    tunnel: w777 -> [w786]
                    shift-right: [w784] -> w776
                    shift-left: w774 -> [w785]
                    tunnel: w775 -> [w779] mode=indexing
                    tunnel: w772 -> [w780]
                    tunnel: w771 -> [w778]
                    i -> [w783]
                    n226 = Greater?(x=w783, y=0) -> (0:w782:bool)
                    n227 = case shown="True" w782 {
                      tunnel: w788 -> [w798 w836]
                      tunnel: w787 -> [w800 _]
                      tunnel: w786 -> [w797 w824]
                      tunnel: w785 -> [w791 w838]
                      tunnel: [w789 w837] -> w784
                      tunnel: w783 -> [_ w834]
                      tunnel: w780 -> [_ w817]
                      tunnel: w779 -> [_ w816]
                      tunnel: w778 -> [_ w804]
                      tunnel: [_ w801] -> _
                      frame False {
                        n228 = Index Array(array=w800, index (row)=w797) -> (element=w799:string[])  [unwired: 1 in]
                        n229 = Index Array(array=w798, index (row)=0 ("索引 (行)")) -> (element=w795:string[])  [unwired: 1 in]
                        n230 = Index Array(array=w795, index=10 ("索引")) -> (element=w792:string)
                        n231 = Replace Array Subset(array=w799, new element=w792, index=4 ("索引")) -> (w790:string[])
                        n232 = Build Array (concatenate)(w791, w790) -> (w789:string[][])
                      }
                      frame True {
                        n233 = Index Array(array=w816, index=0 ("索引")) -> (element=w814:string)
                        n234 = Concatenate Strings("select * from PROP_NUMERICLIMIT where PROP_RESULT=" ("condition"), w814, "" ("字符串")) -> (w821:string)
                        n235 = Increment(x=w824) -> (x+1=w825:i32)
                        n236 = Index Array(array=w836, index (row)=w834) -> (element=w835:string[])  [unwired: 1 in]
                        n237 = Number To Decimal String(number=w834) -> (decimal integer string=w827:string)  [unwired: 1 in]
                        n238 = Number To Decimal String(number=w825) -> (decimal integer string=w829:string)  [unwired: 1 in]
                        n239 = call-poly <vilib>:"DB Tools Execute Query.vi"("error in (no error)"=w804, "SQL query"=w821, "connection reference"=w817) -> ("error out"=w803:errorcluster, "recordset reference"=w818:T4)  [unwired: 5 in]
                        n240 = Index Array(array=w835, index #1=4 ("索引"), index #2=10 ("索引")) -> (element #1=w832:string, element #2=w831:string)
                        n241 = Concatenate Strings(w829, "." ("字符串"), w827) -> (w826:string)
                        n242 = call-poly <vilib>:"DB Tools Fetch Recordset Data.vi"("error in (no error)"=w803, "recordset reference"=w818) -> ("error out"=w802:errorcluster, "recordset data"=w819:variant[][])  [unwired: 3 in, 1 out]
                        n243 = xnode "Database Variant To Data"("database variant"=w819, "error in (no error)"=w802, "type"=string[][] []) -> ("data"=w812:string[][], "error out"=w801:errorcluster)
                        "data 6" <- w812
                        n244 = Index Array(array=w812, index (row)=0 ("索引")) -> (element=w811:string[])  [unwired: 1 in]
                        n245 = Index Array(array=w811, index #1=4 ("索引"), index #2=3 ("索引"), index #3=6 ("索引")) -> (element #1=w807:string, element #2=w806:string, element #3=w805:string)
                        n246 = Build Array(w826, w832, w807, w806, w831, w805) -> (w830:string[])
                        n247 = Build Array (concatenate)(w838, w830) -> (w837:string[][])
                      }
                    }
                  }
                }
              }
            }
            n248 = property on="预览数据" class="MCListbox (strict)"("ItemNames"=w658) -> ()  [unwired: 2 in, 2 out]
          }
          frame True {
          }
        }
      }
      event "保存按钮": Value Change {
        n249 = event-data() -> ("NewVal"=w955:bool)  [unwired: 1 in, 5 out]
        n250 = case shown="True" w955 {
          frame False {
          }
          frame True {
            w957 = "*.csv" ("pattern (all files)")
            n251 = property on="SN" class="Str"() -> ("Value"=w958:string)  [unwired: 2 in, 2 out]
            n252 = call "文件对话框"("start path"=path "D:/", "default name"=w958, "pattern (all files)"=w957, "pattern label"=w957) -> ("selected path"=w959:path)  [unwired: 8 in, 3 out]
            n253 = Not A Number/Path/Refnum?(number/path/refnum=w959) -> (NaN/Path/Refnum?=w960:bool)
            n254 = case shown="False" w960 {
              tunnel: w959 -> [w963 _]
              frame False {
                n255 = property on="预览数据" class="MCListbox (strict)"() -> ("ItemNames"=w964:string[][])  [unwired: 2 in, 2 out]
                n256 = property on="预览数据" class="MCListbox (strict)"() -> ("ColHdrString"=w965:string[])  [unwired: 2 in, 2 out]
                n257 = Build Array (concatenate)(w965, w964) -> (w961:string[][])
                n258 = call-poly <vilib>:"Write Delimited Spreadsheet.vi"("file path (dialog if empty)"=w963, "2D data"=w961, "delimiter (\\t)"="," ("delimiter (\\t)")) -> ()  [unwired: 11 in, 2 out]
              }
              frame True {
              }
            }
          }
        }
      }
      event Panel Close? {
        w969 = TRUE ("Discard?")
        n259 = event-data() -> ()  [unwired: 1 in, 4 out]
        n260 = call <vilib>:"DB Tools Close Connection.vi"("error in (no error)"=w967, "connection reference"=w968) -> ("error out"=→"error out":errorcluster)  [unwired: 5 in]
        n261 = event-data("Discard?"=w969) -> ()  [unwired: 1 in, 1 out]
      }
      event "搜索按钮": Value Change {
        n262 = event-data() -> ("NewVal"=w972:bool)  [unwired: 1 in, 5 out]
        n263 = case shown="False" w972 {
          tunnel: w973 -> [_ w979]
          tunnel: w971 -> [w974 w977]
          tunnel: [w974 w975] -> w970
          frame False {
          }
          frame True {
            n264 = property on="二维码" class="Str"() -> ("Value"=w991:string)  [unwired: 2 in, 2 out]
            n265 = call <vilib>:"Trim Whitespace.vi"("string"=w991) -> ("trimmed string"=w987:string)  [unwired: 1 in]
            n266 = Empty String/Path?(string/path=w987) -> (empty?=w983:bool)
            n267 = Concatenate Strings("select * from UUT_RESULT where UUT_SERIAL_NUMBER=\"" ("condition"), w987, "\"" ("字符串")) -> (w989:string)
            n268 = Select(t="select * from UUT_RESULT" ("condition"), s=w983, f=w989) -> (s? t:f=w985:string)
            n269 = call-poly <vilib>:"DB Tools Execute Query.vi"("error in (no error)"=w977, "SQL query"=w985, "connection reference"=w979) -> ("error out"=w978:errorcluster, "recordset reference"=w990:T4)  [unwired: 5 in]
            n270 = call-poly <vilib>:"DB Tools Fetch Recordset Data.vi"("error in (no error)"=w978, "recordset reference"=w990) -> ("error out"=w976:errorcluster, "recordset data"=w982:variant[][])  [unwired: 3 in, 1 out]
            n271 = xnode "Database Variant To Data"("database variant"=w982, "error in (no error)"=w976, "type"=string[][] [["", " "]]) -> ("data"=w981:string[][], "error out"=w975:errorcluster)
            n272 = property on="筛选结果" class="MCListbox (strict)"("ItemNames"=w981) -> ()  [unwired: 2 in, 2 out]
          }
        }
      }
    }
  }
  n273 = property on="筛选结果" class="MCListbox (strict)"("ItemNames"=w1) -> ()  [unwired: 2 in, 2 out]
  n274 = property on="预览数据" class="MCListbox (strict)"("ItemNames"=w1) -> ()  [unwired: 2 in, 2 out]
  n275 = invoke on="树形" class="Tree (严格)" method="Edit Tree Items.Delete"("Delete Children"=TRUE ("删除子项？")) -> ()  [unwired: 4 in, 5 out]
